vi "Get Summary.vi"(8 "error in (no error)":errorcluster, 10 "Item":string, 11 "Result Model by Reference In":refnum<class "Result Model by Reference.lvclass">) -> (0 "error out":errorcluster, 2 "Summary":string)   [LabVIEW 2020, in "Result Model by Reference.lvclass"]
uses:
  Result Model by Reference.lvclass
  Result Model by Reference.lvclass/Result Model by Reference.ctl
  Result Model/Result Model.lvclass
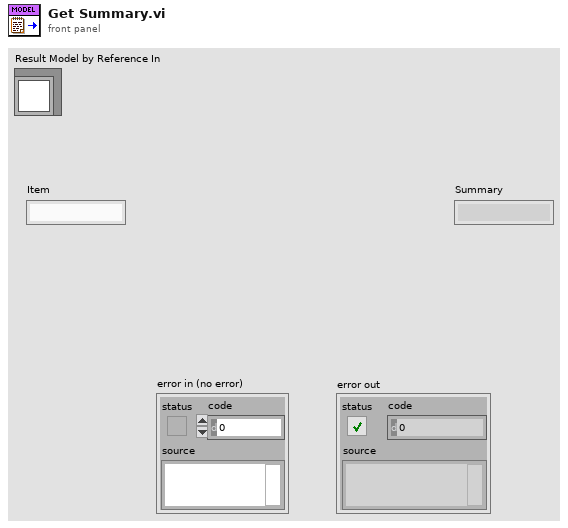
[diagram p1: front panel]
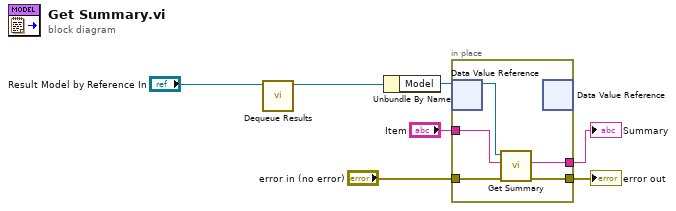
[diagram p0: block diagram]
diagram:
  n1 = call "Dequeue Results.vi"("Result Model by Reference in"="Result Model by Reference In") -> ("Result Model by Reference out"=w1:refnum<class "Result Model by Reference.lvclass">)  [unwired: 10 in]
  n2 = Unbundle By Name(w1) -> ("Model"=w7:refnum<data-value>)
  n3 = in-place {
    in-place-border: "error in (no error)" -> [w12]
    in-place-border: [w11] -> w3
    in-place-border: "Item" -> [w9]
    in-place-border: [w8] -> w2
    n4 = in-place-dvr #1(w7) -> (w10:refnum<class "Result Model.lvclass">)  [unwired: 1 out]
    n5 = call "Get Summary.vi"("error in (no error)"=w12, "Item"=w9, "Result Model In"=w10) -> ("error out"=w11:errorcluster, "Summary"=w8:string)  [unwired: 7 in]
    n6 = in-place-dvr #1() -> ()  [unwired: 1 in, 2 out]
  }
  "Summary" <- w2
  "error out" <- w3
